vi "termo_main__.vi"() -> ()   [LabVIEW 2015]
doc: "Термометрия"
uses:
  <vilib>/NI/Modbus Library/API/Master/Modbus Master.lvclass
  Load and Save Controls_LV2009.llb/RWC_Actions.ctl
  <vilib>/Utility/error.llb/DialogType.ctl
  <vilib>/express/express arith-compare/Formula/XNode/ExpressFormulaBlockNode.xnode
panel:
  in  "счетчик":u16
  out "Связь с блоком":bool
  in  "Tab Control":enum32{"ИЗМЕРЕНИЯ", "НАСТРОЙКИ"}(tab)
  in  "3_ch_visible":bool=TRUE
  out "R2":dbl format="%.2f"
  out "R1":dbl format="%.2f"
  in  "2_ch_visible":bool=TRUE
  in  "1_ch_visible":bool=TRUE
  out "К 2":dbl format="%.2f"
  out "К 1":dbl format="%.2f"
  out "К 3":dbl format="%.2f"
  out "R3":dbl format="%.2f"
  in  "Т min":dbl=4.0 min=-10.0 max=350.0 step=0.1
  in  "Т max":dbl=350.0 min=2.0 max=500.0 step=0.1
  in  "Autoscale":bool=TRUE
  out "сек.":string="0"
  out "часы":string="0"
  in  "Добавить время":dbl(ring)=300.0 items=["10 сек."=10.0, "1 мин."=60.0, "5 мин."=300.0, "20 мин."=1200.0]
  out "мин.":string="1"
  in  "xScale +":bool
  in  "xScale -":bool
  in  "Сохранение в файл":bool
  in  "Buf_size":u16=10 min=1 max=128
  in  "SPS":T1(ring)=enum."5 SPS"
  in  "Пароль":string
  in  "настр. коэфф.":bool caption="Disconn"
  in  "Коэ 2":T2 caption="К 2" {"R0" format="%#_16g"; "k7" format="%#_16g"; "k6" format="%#_16g"; "k5" format="%#_16g"; "k4" format="%#_16g"; "k3" format="%#_16g"; "k2" format="%#_16g"; "k1" format="%#_16g"}
  in  "stop":bool
  in  "Коэ 1":T2 caption="К 1" {"R0" format="%#_16g"; "k7" format="%#_16g"; "k6" format="%#_16g"; "k5" format="%#_16g"; "k4" format="%#_16g"; "k3" format="%#_16g"; "k2" format="%#_16g"; "k1" format="%#_16g"}
  in  "GraphLookB":bool
  in  "IP":string
  in  "Порт":u16
  in  "Коэ 3":T2 caption="К 3" {"R0" format="%#_16g"; "k7" format="%#_16g"; "k6" format="%#_16g"; "k5" format="%#_16g"; "k4" format="%#_16g"; "k3" format="%#_16g"; "k2" format="%#_16g"; "k1" format="%#_16g"}
  out "Path":string
  in  "интервал сохр.":u16=10 min=1 max=3600 step=1
  out "Сутки":string
  in  "Запись в файл":bool
  out "File header exist?":bool caption="Disconn"
  in  "ADC_dyn_range":T3(ring)=enum."± 0.625 В"
  out "refnum out":refnum<file>
  out "Graphs T":dynamicdata(graph) caption="ТЕМПЕРАТУРА, К"
  out "Связь":refnum<class "Modbus Master.lvclass">
  in  "Buf_size":u8=1 min=1 max=128
  in  "SPS":T1(ring)
  out "Расположение файла":path
  # "Т [K]"
  # "R [Ом]"
  # ":"
  # ":"
  # "Шкала Т"
  # "id 100"
  # "Скорость измерений"
  # "Размер буфера усредн."
  # "SPS = Samples Per Second"
  # "сек."
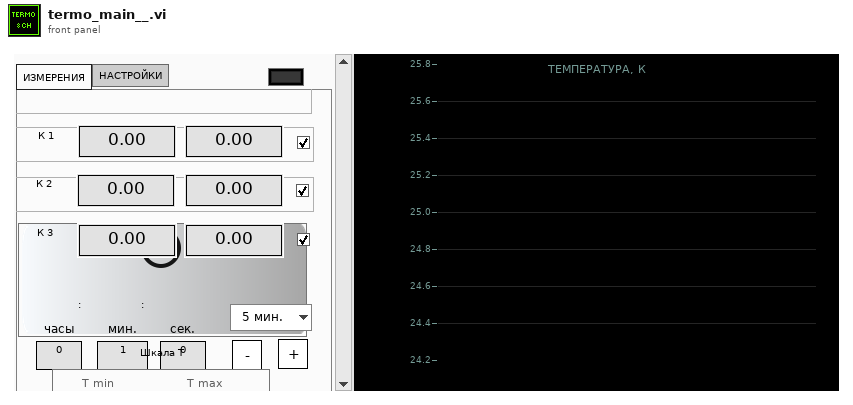
[diagram p1: front panel]
types:
  T1 = enum16{"2,5 SPS", "5 SPS", "10 SPS", "25 SPS", "50 SPS", "100 SPS", "500 SPS", "1 kSPS"}
  T2 = cluster{"k1":ext, "k2":ext, "k3":ext, "k4":ext, "k5":ext, "k6":ext, "k7":ext, "R0":ext}
  T3 = enum16{"± 5 В", "± 2.5 В", "± 1.25 В", "± 0.625 В", "± 312.5 мВ", "± 156.25 мВ", "± 78.125 мВ"}
  T4 = typedef "DialogType.ctl" = u16
  T5 = typedef "RWC_Actions.ctl" = enum16{"Read", "Write", "Read and Create"}
  T6 = enum8{"Enabled", "Disabled", "Disabled and Grayed Out"}
  T7 = typedef "LVDateTimeRec.ctl" = cluster{"fractional second":dbl, "second":i32, "minute":i32, "hour":i32, "day of month":i32, "month":i32, "year":i32, "day of week":i32, "day of year":i32, "DST":i32}
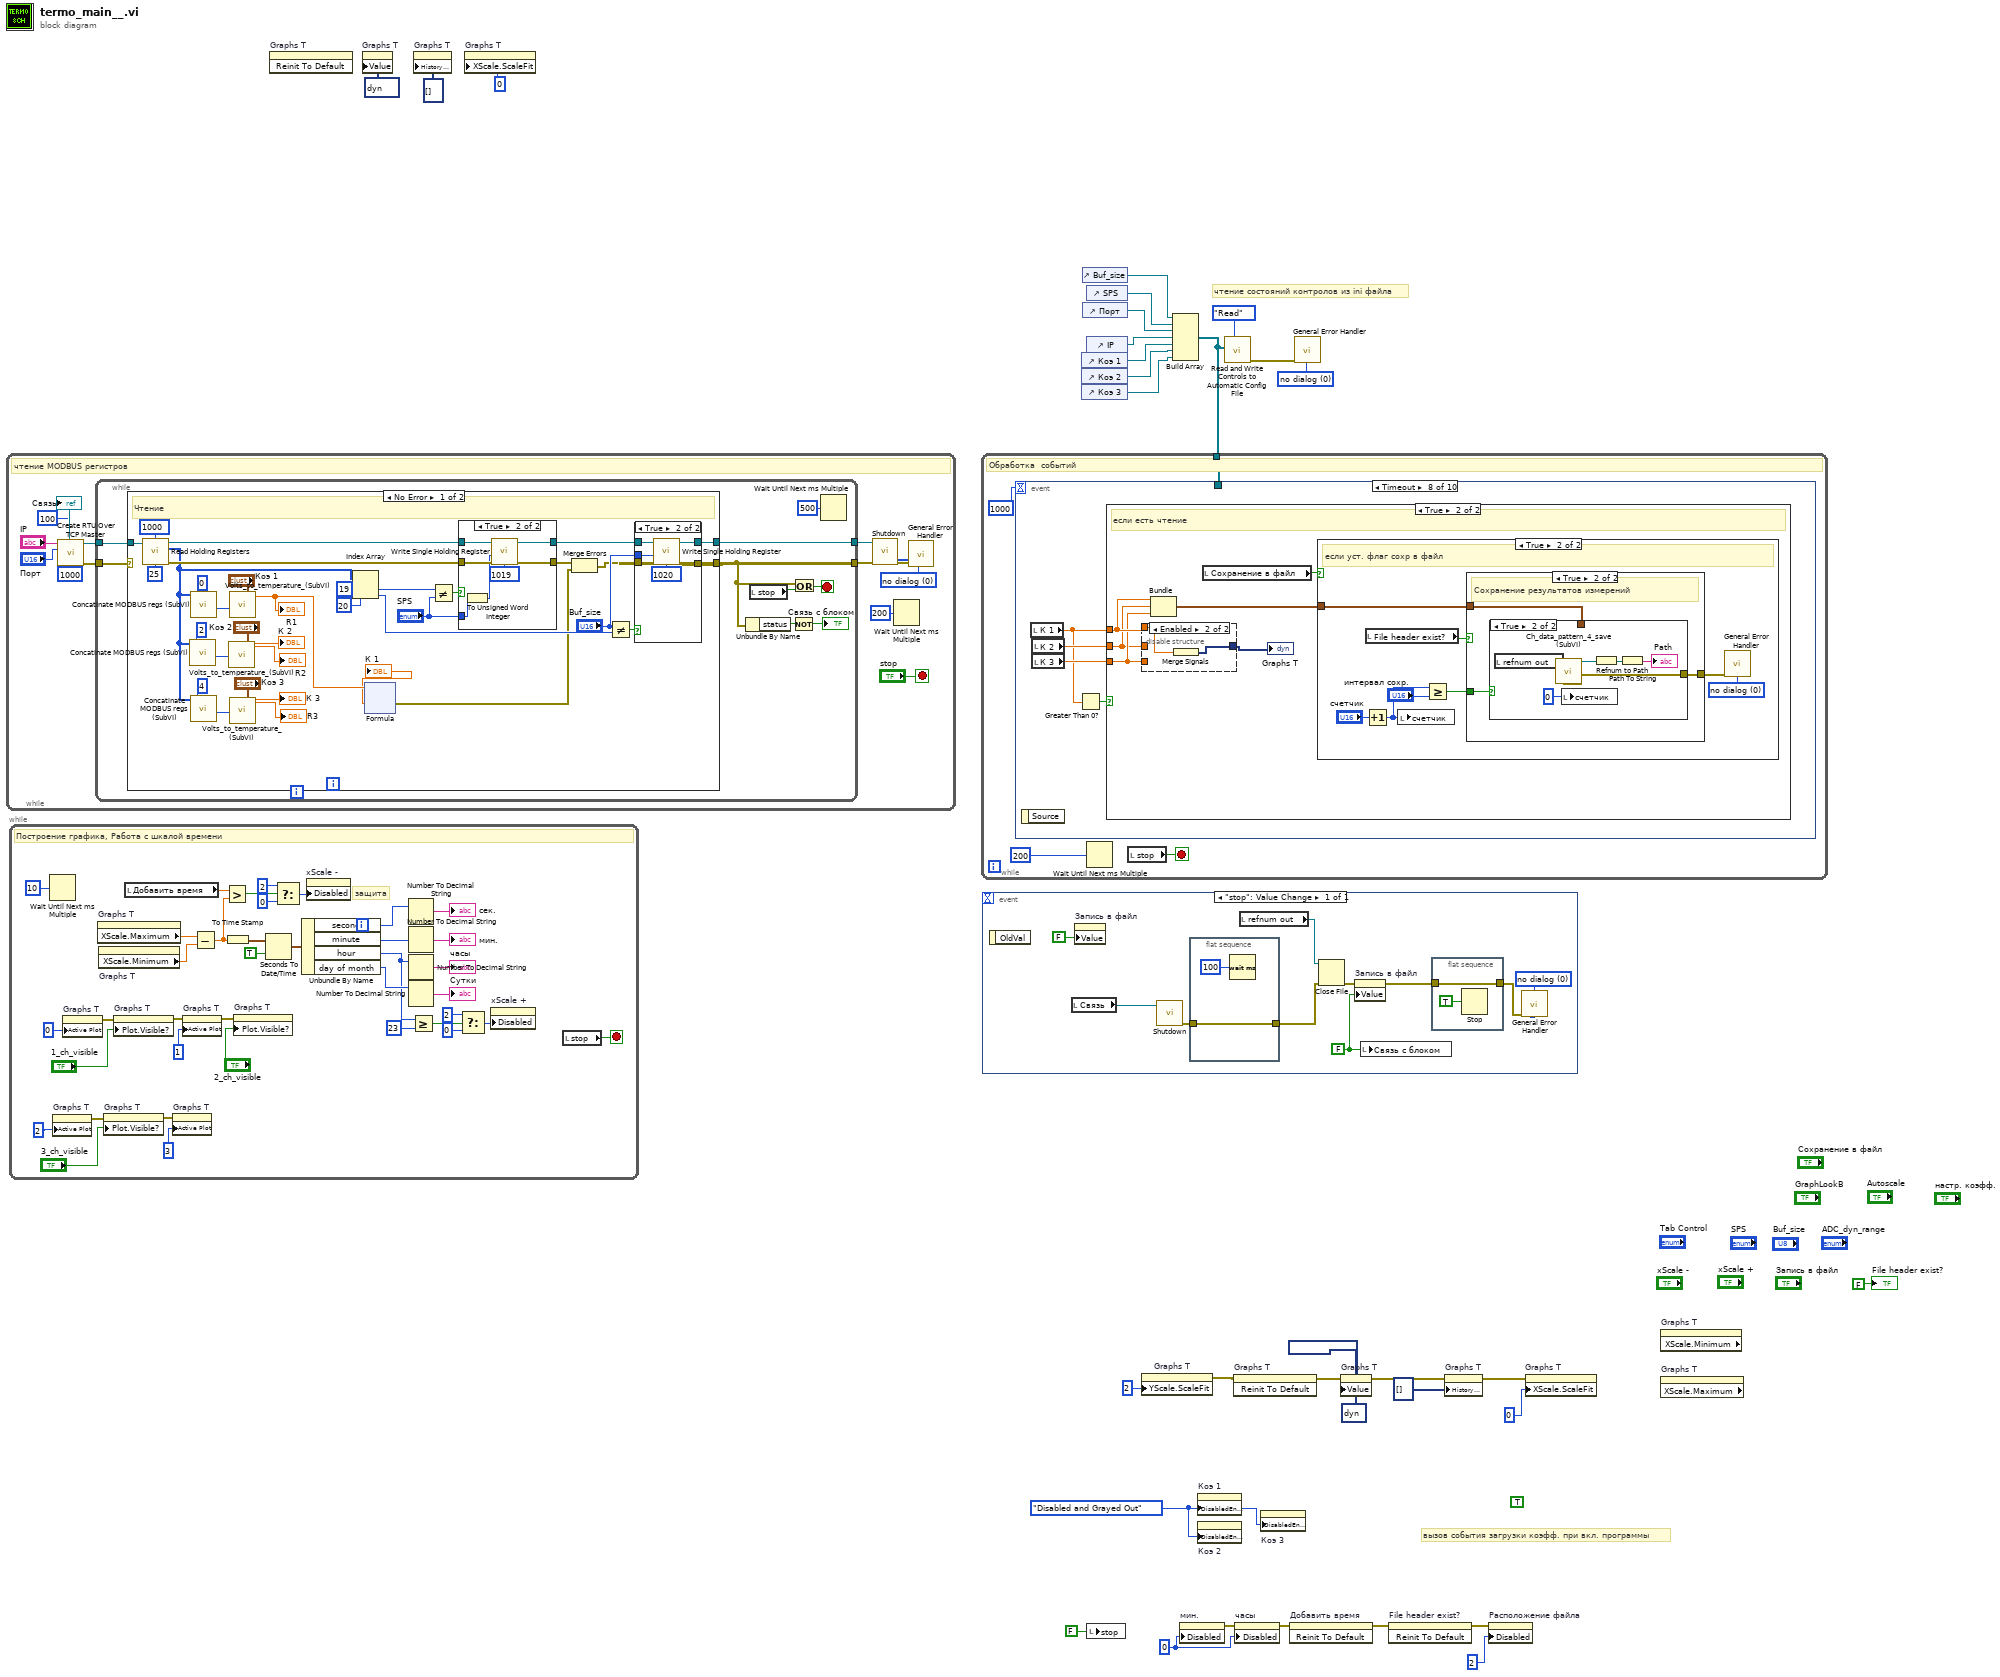
[diagram p0: block diagram]
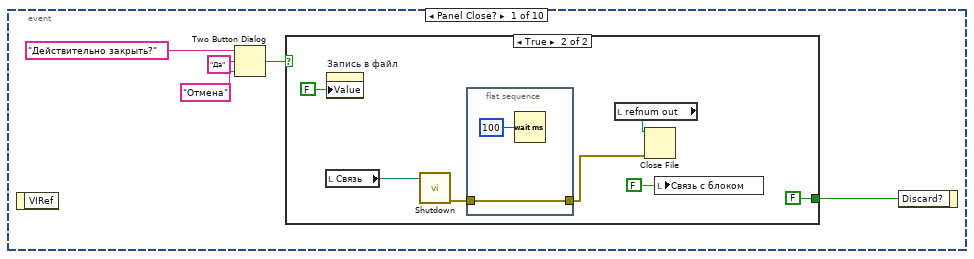
[diagram p2: hidden frame]
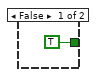
[diagram p3: hidden frame]
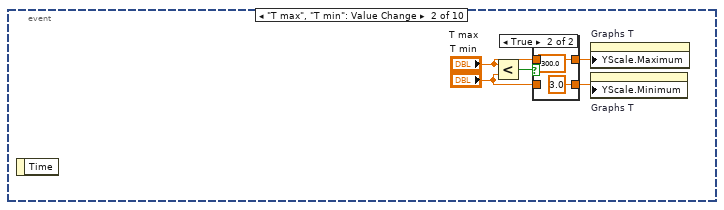
[diagram p4: hidden frame]
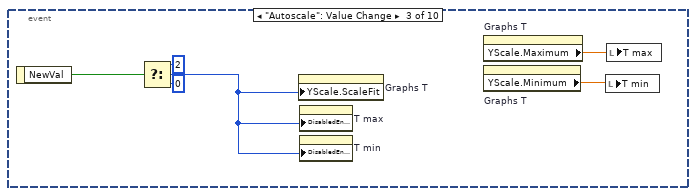
[diagram p6: hidden frame]
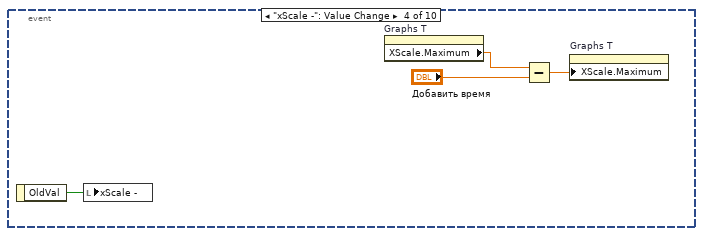
[diagram p7: hidden frame]
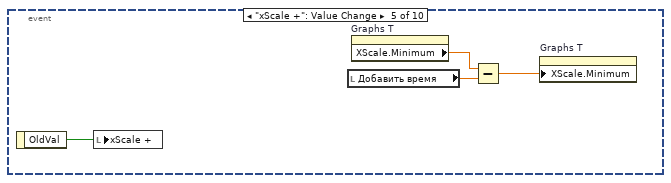
[diagram p8: hidden frame]
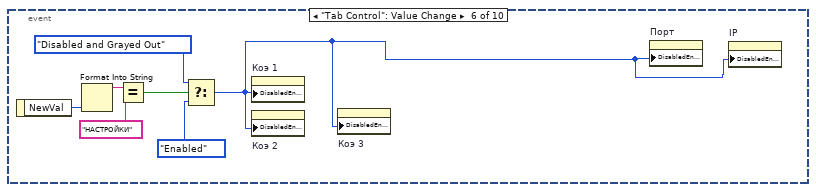
[diagram p9: hidden frame]
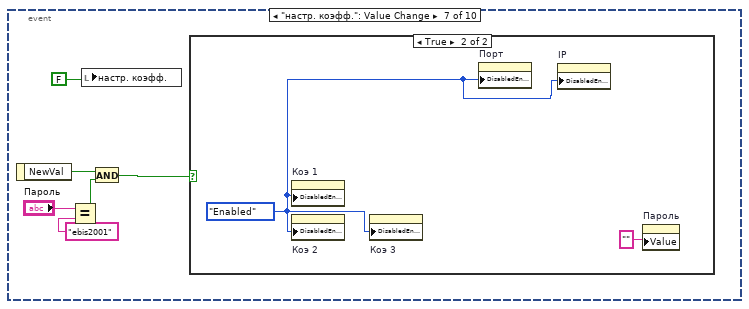
[diagram p10: hidden frame]
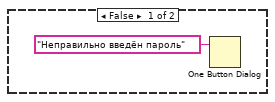
[diagram p11: hidden frame]
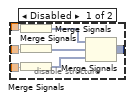
[diagram p13: hidden frame]
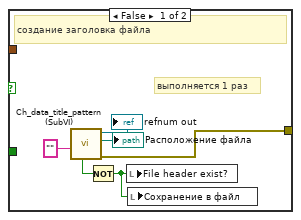
[diagram p15: hidden frame]
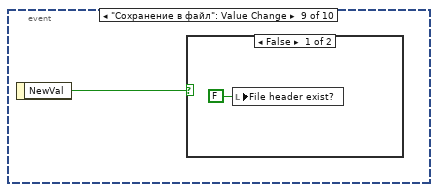
[diagram p17: hidden frame]
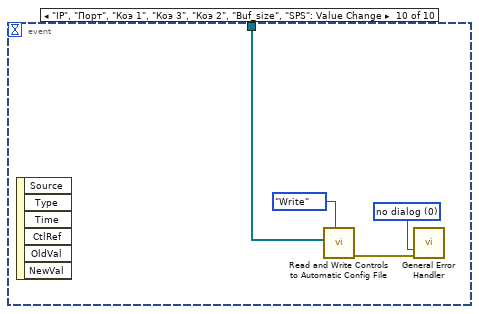
[diagram p19: hidden frame]
diagram:
  w12 = T4 0 items=["no dialog", "OK message", "continue or stop message", "OK message + warnings", "continue/stop + warnings"] ("type of dialog (OK msg:1)")
  (unwired) TRUE ("Value (Signaling)")
  w15 = T6."Disabled and Grayed Out" ("Disabled")
  w30 = u8 0 ("Disabled")
  # "чтение состояний контролов из ini файла"
  # "вызов события загрузки коэфф. при вкл. программы"
  n1 = while {
    stop <- "stop" stop-if-true
    w33 = T4 0 items=["no dialog", "OK message", "continue or stop message", "OK message + warnings", "continue/stop + warnings"] ("type of dialog (OK msg:1)")
    # "чтение MODBUS регистров"
    n2 = call "Create RTU Over TCP Master.vi"("unit ID"=u8 100, "connect timeout ms"=1000, "port (502)"="Порт", "address"="IP") -> ("error out"=w37:errorcluster, "TCP master instance"=w38:refnum<class "Modbus Master.lvclass">)  [unwired: 6 in]
    "Связь" <- w38
    n3 = while {
      tunnel: w38 -> [w52]
      tunnel: w37 -> [w51]
      tunnel: [w45] -> w36
      tunnel: [w50] -> w35
      stop <- w48 stop-if-true
      n4 = case shown="No Error" w51 {
        selector: w51 -> [_ w117]
        tunnel: w52 -> [w85 w118]
        tunnel: [w69 w117] -> w45
        tunnel: [w70 w118] -> w50
        frame No Error {
          # "Чтение"
          n5 = call-dynamic "Read Holding Registers.vi"("number of inputs"=u16 25, "starting address"=u16 1000, "Modbus master in"=w85) -> ("error out"=w67:errorcluster, "register values"=w66:u16[], "Modbus master out"=w68:refnum<class "Modbus Master.lvclass">)  [unwired: 6 in]
          n6 = call "Concatinate MODBUS regs (SubVI).vi"("LSB reg num"=u16 2, "registers array in"=w66) -> ("register data"=w80:i32)  [unwired: 8 in, 1 out]
          n7 = call "Concatinate MODBUS regs (SubVI).vi"("LSB reg num"=u16 0, "registers array in"=w66) -> ("register data"=w82:i32)  [unwired: 8 in, 1 out]
          n8 = call "Concatinate MODBUS regs (SubVI).vi"("LSB reg num"=u16 4, "registers array in"=w66) -> ("register data"=w73:i32)  [unwired: 8 in, 1 out]
          n9 = call "Volts_to_temperature_(SubVI).vi"("Resistance"=w80, "koeff. cluster"="Коэ 2") -> ("T solvation"=→"К 2":dbl, "meas_voltage"=→"R2":dbl)  [unwired: 21 in, 3 out]
          n10 = call "Volts_to_temperature_(SubVI).vi"("Resistance"=w82, "koeff. cluster"="Коэ 1") -> ("meas_voltage"=w57:dbl)  [unwired: 21 in, 4 out]
          "R1" <- w57
          n11 = call "Volts_to_temperature_(SubVI).vi"("Resistance"=w73, "koeff. cluster"="Коэ 3") -> ("T solvation"=→"К 3":dbl, "meas_voltage"=→"R3":dbl)  [unwired: 21 in, 3 out]
          n12 = Index Array(array=w66, index #1=19 ("index"), index #2=20 ("index")) -> (element #1=w65:u16, element #2=w59:u16)
          n13 = xnode "Formula"("R"=w57) -> ("Result"=→"К 1":ext, "error out"=w53:errorcluster)  [unwired: 2 in]
          n14 = Not Equal?(x=w65, y="SPS") -> (x != y?=w64:bool)
          n15 = case shown="True" w64 {
            tunnel: w68 -> [w107 w114]
            tunnel: w67 -> [w106 w113]
            tunnel: [w107 w111] -> w71
            tunnel: [w106 w110] -> w55
            tunnel: "SPS" -> [_ w109]
            frame False {
            }
            frame True {
              n16 = To Unsigned Word Integer(number=w109) -> (unsigned 16bit integer=w108:u16)
              n17 = call-dynamic "Write Single Holding Register.vi"("error in"=w113, "register to write"=w108, "address"=u16 1019 ("starting address"), "Modbus master in"=w114) -> ("error out"=w110:errorcluster, "Modbus master out"=w111:refnum<class "Modbus Master.lvclass">)  [unwired: 6 in]
            }
          }
          n18 = Merge Errors(w55, w53) -> (w54:errorcluster)
          n19 = Not Equal?(x="Buf_size", y=w59) -> (x != y?=w60:bool)
          n20 = case shown="True" w60 {
            tunnel: w71 -> [w99 w105]
            tunnel: w54 -> [w98 w104]
            tunnel: [w99 w102] -> w70
            tunnel: [w98 w101] -> w69
            tunnel: "Buf_size" -> [_ w100]
            frame False {
            }
            frame True {
              n21 = call-dynamic "Write Single Holding Register.vi"("error in"=w104, "register to write"=w100, "address"=u16 1020 ("starting address"), "Modbus master in"=w105) -> ("error out"=w101:errorcluster, "Modbus master out"=w102:refnum<class "Modbus Master.lvclass">)  [unwired: 6 in]
            }
          }
        }
        frame Error {
          w115 = -1.0 ("R1")
          w116 = -1.0 ("R1")
          n22 = local write "R1"(w115) -> ()
          n23 = local write "R2"(w115) -> ()
          n24 = local write "R3"(w115) -> ()
          n25 = local write "К 1"(w116) -> ()
          n26 = local write "К 3"(w116) -> ()
          n27 = local write "К 2"(w116) -> ()
        }
      }
      n28 = Unbundle By Name(w45) -> ("status"=w47:bool)
      n29 = local read "stop"() -> (w49:bool)
      n30 = Not(x=w47) -> (.not. x?=→"Связь с блоком":bool)
      n31 = Or(x=w45, y=w49) -> (x .or. y?=w48:bool)
      n32 = Wait Until Next ms Multiple(millisecond multiple=u32 500) -> ()  [unwired: 1 out]
    }
    n33 = call-dynamic "Shutdown.vi"("error in"=w36, "Modbus master in"=w35) -> ("error out"=w34:errorcluster)  [unwired: 9 in]
    n34 = Wait Until Next ms Multiple(millisecond multiple=u32 200) -> ()  [unwired: 1 out]
    n35 = call <vilib>:"General Error Handler.vi"("type of dialog (OK msg:1)"=w33, "error in (no error)"=w34) -> ()  [unwired: 1 in, 13 out]
  }
  n36 = while {
    stop <- w156 stop-if-true
    # "защита"
    # "Построение графика, Работа с шкалой времени"
    n37 = Wait Until Next ms Multiple(millisecond multiple=u32 10) -> ()  [unwired: 1 out]
    n38 = property on="Graphs T" class="WFChart (strict)"("Active Plot"=u32 2) -> (error out=w123:errorcluster)  [unwired: 2 in, 1 out]
    n39 = property on="Graphs T" class="WFChart (strict)"("Active Plot"=u32 0) -> (error out=w124:errorcluster)  [unwired: 2 in, 1 out]
    n40 = property on="Graphs T" class="WFChart (strict)"() -> ("XScale.Maximum"=w132:dbl)  [unwired: 2 in, 2 out]
    n41 = property on="Graphs T" class="WFChart (strict)"() -> ("XScale.Minimum"=w131:dbl)  [unwired: 2 in, 2 out]
    n42 = property on="Graphs T" class="WFChart (strict)"(error in=w123, "Plot.Visible?"="3_ch_visible") -> (error out=w119:errorcluster)  [unwired: 1 in, 1 out]
    n43 = property on="Graphs T" class="WFChart (strict)"(error in=w124, "Plot.Visible?"="1_ch_visible") -> (error out=w129:errorcluster)  [unwired: 1 in, 1 out]
    n44 = local read "Добавить время"() -> (w155:dbl)
    n45 = property on="Graphs T" class="WFChart (strict)"(error in=w119, "Active Plot"=u32 3) -> ()  [unwired: 1 in, 2 out]
    n46 = property on="Graphs T" class="WFChart (strict)"(error in=w129, "Active Plot"=u32 1) -> (error out=w127:errorcluster)  [unwired: 1 in, 1 out]
    n47 = Subtract(x=w132, y=w131) -> (x-y=w145:dbl)
    n48 = Greater?(x=w155, y=w145) -> (0:w138:bool)
    n49 = To Time Stamp(1:w145) -> (0:w153:timestamp)
    n50 = property on="Graphs T" class="WFChart (strict)"(error in=w127, "Plot.Visible?"="2_ch_visible") -> ()  [unwired: 1 in, 2 out]
    n51 = Seconds To Date/Time(time stamp (now)=w153, to UTC (F)=TRUE) -> (date time rec=w152:T7)
    n52 = Select(t=u8 2 ("Disabled"), s=w138, f=u8 0 ("Disabled")) -> (s? t:f=w141:u8)
    n53 = Unbundle By Name(w152) -> ("second"=w151:i32, "minute"=w150:i32, "hour"=w143:i32, "day of month"=w149:i32)
    n54 = property on="xScale -" class="Bool (strict)"("Disabled"=w141) -> ()  [unwired: 2 in, 2 out]
    n55 = Number To Decimal String(number=w151) -> (decimal integer string=→"сек.":string)  [unwired: 1 out]
    n56 = Number To Decimal String(number=w150) -> (decimal integer string=→"мин.":string)  [unwired: 1 out]
    n57 = Number To Decimal String(number=w143) -> (decimal integer string=→"часы":string)  [unwired: 1 out]
    n58 = Number To Decimal String(number=w149) -> (decimal integer string=→"Сутки":string)  [unwired: 1 out]
    n59 = Greater Or Equal?(x=w143, y=23) -> (x >= y?=w134:bool)
    n60 = Select(t=u8 2 ("Disabled"), s=w134, f=u8 0 ("Disabled")) -> (s? t:f=w137:u8)
    n61 = property on="xScale +" class="Bool (strict)"("Disabled"=w137) -> ()  [unwired: 2 in, 2 out]
    n62 = local read "stop"() -> (w156:bool)
  }
  n63 = invoke on="Graphs T" class="WFChart (strict)" method="Reinit To Default"() -> ()  [unwired: 3 in, 3 out]
  n64 = property on="Graphs T" class="WFChart (strict)"("Value"=dynamicdata [{"t0"=timestamp(3465273261.7246556 s since 1904-01-01), "dt"=1.0, "Y"=[0.1931097262457384]}, {"t0"=timestamp(3465273261.7246556 s since 1904-01-01), "dt"=1.0, "Y"=[0.3594116459482981]}, {"t0"=timestamp(3465273261.7246556 s since 1904-01-01), "dt"=1.0, "Y"=[0.8898205452798131]}, {"t0"=timestamp(3465273261.7246556 s since 1904-01-01), "dt"=1.0, "Y"=[0.747699236883661]}] ("Graphs")) -> ()  [unwired: 2 in, 2 out]
  n65 = property on="Graphs T" class="WFChart (strict)"("History Data"=dynamicdata[] []) -> ()  [unwired: 2 in, 2 out]
  n66 = property on="Graphs T" class="WFChart (strict)"("XScale.ScaleFit"=u8 0 ("Y Scale.Scale Fit")) -> ()  [unwired: 2 in, 2 out]
  n67 = event shown="[0] \"stop\": Value Change" {
    selector: _ -> [_]
    dyn-events: _ -> [_]
    timeout: _ -> [_]
    event "stop": Value Change {
      w160 = T4 0 items=["no dialog", "OK message", "continue or stop message", "OK message + warnings", "continue/stop + warnings"] ("type of dialog (OK msg:1)")
      w157 = FALSE ("Запись в файл")
      n68 = event-data() -> ()  [unwired: 1 in, 1 out]
      n69 = local read "Связь"() -> (w162:refnum<class "Modbus Master.lvclass">)
      n70 = property on="Запись в файл" class="Bool (strict)"("Value"=FALSE ("Запись в файл")) -> ()  [unwired: 2 in, 2 out]
      n71 = call-dynamic "Shutdown.vi"("Modbus master in"=w162) -> ("error out"=w161:errorcluster)  [unwired: 10 in]
      n72 = flat-sequence {
        tunnel: w161 -> [w169]
        tunnel: [w169] -> w158
        frame #0 {
          n73 = Wait (ms)(milliseconds to wait=u32 100) -> ()  [unwired: 1 out]
        }
      }
      n74 = local read "refnum out"() -> (w165:refnum<file>)
      n75 = Close File(refnum=w165, error in=w158) -> (error out=w164:errorcluster)  [unwired: 1 out]
      n76 = property on="Запись в файл" class="Bool (strict)"(error in=w164, "Value"=w157) -> (error out=w163:errorcluster)  [unwired: 1 in, 1 out]
      n77 = local write "Связь с блоком"(w157) -> ()
      n78 = flat-sequence {
        tunnel: w163 -> [w168]
        tunnel: [w168] -> w159
        frame #0 {
          n79 = Stop(stop? (T)=TRUE) -> ()
        }
      }
      n80 = call <vilib>:"General Error Handler.vi"("error in (no error)"=w159, "[exception action] (none:0)"=w160) -> ()  [unwired: 2 in, 12 out]
    }
  }
  n81 = control-ref of="Коэ 1"() -> (w6:refnum<vi>)
  n82 = control-ref of="Коэ 2"() -> (w5:refnum<vi>)
  n83 = control-ref of="Коэ 3"() -> (w4:refnum<vi>)
  n84 = control-ref of="Buf_size"() -> (w8:refnum<vi>)
  n85 = control-ref of="Порт"() -> (w11:refnum<vi>)
  n86 = control-ref of="SPS"() -> (w9:refnum<vi>)
  n87 = control-ref of="IP"() -> (w7:refnum<vi>)
  n88 = local write "stop"(FALSE ("Boolean")) -> ()
  n89 = property on="Graphs T" class="WFChart (strict)"("YScale.ScaleFit"=u8 2 ("Y Scale.Scale Fit")) -> (error out=w23:errorcluster)  [unwired: 2 in, 1 out]
  n90 = Build Array(w8, w9, w11, w7, w6, w5, w4) -> (w10:refnum<vi>[])
  n91 = while {
    tunnel: w10 -> [w171]
    stop <- w173 stop-if-true
    # "Обработка  событий"
    n92 = event shown="[7] Timeout" {
      selector: _ -> [_ _ _ _ _ _ _ _ _ _]
      dyn-events: _ -> [_ _ _ _ _ _ _ _ _ _]
      timeout: 1000 -> [_ _ _ _ _ _ _ _ _ _]
      tunnel: w171 -> [_ _ _ _ _ _ _ _ _ w272]
      event Panel Close? {
        n93 = event-data() -> ()  [unwired: 2 out]
        n94 = Two Button Dialog(message="Действительно закрыть?", 1:"Отмена" ("T button name (\"OK\")"), 2:"Да" ("T button name (\"OK\")")) -> (T button?=w179:bool)
        n95 = case shown="True" w179 {
          tunnel: [TRUE ("Discard?") FALSE ("Discard?")] -> w175
          frame False {
          }
          frame True {
            n96 = local read "Связь"() -> (w184:refnum<class "Modbus Master.lvclass">)
            n97 = property on="Запись в файл" class="Bool (strict)"("Value"=FALSE ("Запись в файл")) -> ()  [unwired: 2 in, 2 out]
            n98 = call-dynamic "Shutdown.vi"("Modbus master in"=w184) -> ("error out"=w183:errorcluster)  [unwired: 10 in]
            n99 = flat-sequence {
              tunnel: w183 -> [w188]
              tunnel: [w188] -> w182
              frame #0 {
                n100 = Wait (ms)(milliseconds to wait=u32 100) -> ()  [unwired: 1 out]
              }
            }
            n101 = local read "refnum out"() -> (w186:refnum<file>)
            n102 = Close File(refnum=w186, error in=w182) -> ()  [unwired: 2 out]
            n103 = local write "Связь с блоком"(FALSE ("Связь с блоком 4")) -> ()
          }
        }
        n104 = event-data("Discard?"=w175) -> ()  [unwired: 1 in, 1 out]
      }
      event "Т max", "Т min": Value Change {
        n105 = event-data() -> ()  [unwired: 2 out]
        n106 = Less?(x="Т max", y="Т min") -> (x < y?=w194:bool)
        n107 = case shown="True" w194 {
          tunnel: [w195 300.0 ("x+1")] -> w192
          tunnel: [w196 3.0 ("x+1")] -> w193
          tunnel: "Т max" -> [w195 _]
          tunnel: "Т min" -> [w196 _]
          frame False {
          }
          frame True {
          }
        }
        n108 = property on="Graphs T" class="WFChart (strict)"("YScale.Maximum"=w192) -> ()  [unwired: 2 in, 2 out]
        n109 = property on="Graphs T" class="WFChart (strict)"("YScale.Minimum"=w193) -> ()  [unwired: 2 in, 2 out]
      }
      event "Autoscale": Value Change {
        n110 = event-data() -> ("NewVal"=w199:bool)  [unwired: 1 out]
        n111 = Select(t=u8 2 ("Y Scale.Scale Fit"), s=w199, f=u8 0 ("Y Scale.Scale Fit")) -> (s? t:f=w202:u8)
        n112 = property on="Graphs T" class="WFChart (strict)"("YScale.ScaleFit"=w202) -> ()  [unwired: 2 in, 2 out]
        n113 = property on="Т max" class="DigNum (strict)"("DisabledEnum"=w202) -> ()  [unwired: 2 in, 2 out]
        n114 = property on="Т min" class="DigNum (strict)"("DisabledEnum"=w202) -> ()  [unwired: 2 in, 2 out]
        n115 = property on="Graphs T" class="WFChart (strict)"() -> ("YScale.Maximum"=w204:dbl)  [unwired: 2 in, 2 out]
        n116 = property on="Graphs T" class="WFChart (strict)"() -> ("YScale.Minimum"=w203:dbl)  [unwired: 2 in, 2 out]
        n117 = local write "Т min"(w203) -> ()
        n118 = local write "Т max"(w204) -> ()
      }
      event "xScale -": Value Change {
        n119 = event-data() -> ("OldVal"=w208:bool)  [unwired: 1 out]
        n120 = local write "xScale -"(w208) -> ()
        n121 = property on="Graphs T" class="WFChart (strict)"() -> ("XScale.Maximum"=w206:dbl)  [unwired: 2 in, 2 out]
        n122 = Subtract(x=w206, y="Добавить время") -> (x-y=w205:dbl)
        n123 = property on="Graphs T" class="WFChart (strict)"("XScale.Maximum"=w205) -> ()  [unwired: 2 in, 2 out]
      }
      event "xScale +": Value Change {
        n124 = event-data() -> ("OldVal"=w212:bool)  [unwired: 1 out]
        n125 = local write "xScale +"(w212) -> ()
        n126 = local read "Добавить время"() -> (w211:dbl)
        n127 = property on="Graphs T" class="WFChart (strict)"() -> ("XScale.Minimum"=w210:dbl)  [unwired: 2 in, 2 out]
        n128 = Subtract(x=w210, y=w211) -> (x-y=w209:dbl)
        n129 = property on="Graphs T" class="WFChart (strict)"("XScale.Minimum"=w209) -> ()  [unwired: 2 in, 2 out]
      }
      event "Tab Control": Value Change {
        n130 = event-data() -> ("NewVal"=w219:enum32{"ИЗМЕРЕНИЯ", "НАСТРОЙКИ"})  [unwired: 1 out]
        n131 = Format Into String(w219) -> (resulting string=w218:string)  [unwired: 3 in, 1 out]
        n132 = Equal?(x=w218, y="НАСТРОЙКИ") -> (x = y?=w216:bool)
        n133 = Select(t=T6."Disabled and Grayed Out" ("Disabled"), s=w216, f=T6."Enabled" ("Disabled")) -> (s? t:f=w213:T6)
        n134 = property on="Коэ 1" class="Clust (strict)"("DisabledEnum"=w213) -> ()  [unwired: 2 in, 2 out]
        n135 = property on="Коэ 2" class="Clust (strict)"("DisabledEnum"=w213) -> ()  [unwired: 2 in, 2 out]
        n136 = property on="Коэ 3" class="Clust (strict)"("DisabledEnum"=w213) -> ()  [unwired: 2 in, 2 out]
        n137 = property on="Порт" class="DigNum (strict)"("DisabledEnum"=w213) -> ()  [unwired: 2 in, 2 out]
        n138 = property on="IP" class="Str"("DisabledEnum"=w213) -> ()  [unwired: 2 in, 2 out]
      }
      event "настр. коэфф.": Value Change {
        n139 = event-data() -> ("NewVal"=w225:bool)  [unwired: 1 out]
        n140 = Equal?(x="Пароль", y="ebis2001") -> (x = y?=w222:bool)
        n141 = local write "настр. коэфф."(FALSE ("насстр. коэфф.")) -> ()
        n142 = And(x=w225, y=w222) -> (x .and. y?=w221:bool)
        n143 = case shown="True" w221 {
          frame False {
            n144 = One Button Dialog(message="Неправильно введён пароль") -> ()  [unwired: 1 in, 1 out]
          }
          frame True {
            w227 = T6."Enabled" ("Disabled")
            n145 = property on="Коэ 1" class="Clust (strict)"("DisabledEnum"=w227) -> ()  [unwired: 2 in, 2 out]
            n146 = property on="Коэ 2" class="Clust (strict)"("DisabledEnum"=w227) -> ()  [unwired: 2 in, 2 out]
            n147 = property on="Коэ 3" class="Clust (strict)"("DisabledEnum"=w227) -> ()  [unwired: 2 in, 2 out]
            n148 = property on="Порт" class="DigNum (strict)"("DisabledEnum"=w227) -> ()  [unwired: 2 in, 2 out]
            n149 = property on="IP" class="Str"("DisabledEnum"=w227) -> ()  [unwired: 2 in, 2 out]
            n150 = property on="Пароль" class="Str"("Value"="" ("Пароль")) -> ()  [unwired: 2 in, 2 out]
          }
        }
      }
      event Timeout {
        n151 = event-data() -> ()  [unwired: 2 out]
        n152 = local read "К 1"() -> (w229:dbl)
        n153 = local read "К 2"() -> (w232:dbl)
        n154 = local read "К 3"() -> (w230:dbl)
        n155 = Greater Than 0?(x=w229) -> (x > 0?=w231:bool)
        n156 = case shown="True" w231 {
          tunnel: w229 -> [_ w237]
          tunnel: w230 -> [_ w236]
          tunnel: w232 -> [_ w234]
          frame False {
          }
          frame True {
            # "если есть чтение"
            n157 = disable-structure shown="Enabled" {
              disable-tunnel: [w242 w246] -> w238
              disable-tunnel: w237 -> [w241 w247]
              disable-tunnel: w236 -> [w240 _]
              disable-tunnel: w234 -> [w239 _]
              frame Disabled {
                n158 = Merge Signals(w241) -> (w245:dynamicdata)
                n159 = Merge Signals(w239) -> (w244:dynamicdata)
                n160 = Merge Signals(w240) -> (w243:dynamicdata)
                n161 = Merge Signals(w245, w244, w243) -> (w242:dynamicdata)
              }
              frame Enabled {
                n162 = Merge Signals(w247) -> (w246:dynamicdata)
              }
            }
            "Graphs T" <- w238
            n163 = Bundle("К 1"=w237, "К 2"=w234, "К 3"=w236) -> (w235:cluster{"К 1":dbl, "К 2":dbl, "К 3":dbl})  [unwired: 1 in]
            n164 = local read "Сохранение в файл"() -> (w233:bool)
            n165 = case shown="True" w233 {
              tunnel: w235 -> [_ w255]
              frame False {
              }
              frame True {
                w254 = T4 0 items=["no dialog", "OK message", "continue or stop message", "OK message + warnings", "continue/stop + warnings"] ("type of dialog (OK msg:1)")
                # "если уст. флаг сохр в файл"
                n166 = Increment(x="счетчик") -> (x+1=w251:u16)
                n167 = local read "File header exist?"() -> (w249:bool)
                n168 = local write "счетчик"(w251) -> ()
                n169 = Greater Or Equal?(x=w251, y="интервал сохр.") -> (x >= y?=w250:bool)
                n170 = case shown="True" w249 {
                  tunnel: w255 -> [_ w264]
                  tunnel: [w258 w263] -> w253
                  tunnel: w250 -> [_ w262]
                  frame False {
                    # "выполняется 1 раз"
                    # "создание заголовка файла"
                    n171 = call "Ch_data_title_pattern (SubVI).vi"("Единица измерений"="") -> ("error out"=w258:errorcluster, "Path"=→"Расположение файла":path, "Byte Stream File out"=→"refnum out":refnum<file>, "cancelled"=w257:bool)  [unwired: 7 in]
                    n172 = Not(x=w257) -> (.not. x?=w256:bool)
                    n173 = local write "File header exist?"(w256) -> ()
                    n174 = local write "Сохранение в файл"(w256) -> ()
                  }
                  frame True {
                    # "Сохранение результатов измерений"
                    n175 = case shown="True" w262 {
                      tunnel: w264 -> [_ _]
                      tunnel: [_ w265] -> w263
                      frame False {
                      }
                      frame True {
                        n176 = local read "refnum out"() -> (w269:refnum<file>)
                        n177 = call "Ch_data_pattern_4_save (SubVI).vi"() -> ("error out"=w265:errorcluster)  [unwired: 27 in]
                        n178 = local write "счетчик"(u8 0 ("счетчик")) -> ()
                        n179 = Refnum to Path(1:w269) -> (0:w268:path)
                        n180 = Path To String(path=w268) -> (string=→"Path":string)
                      }
                    }
                  }
                }
                n181 = call <vilib>:"General Error Handler.vi"("type of dialog (OK msg:1)"=w254, "error in (no error)"=w253) -> ()  [unwired: 1 in, 13 out]
              }
            }
          }
        }
      }
      event "Сохранение в файл": Value Change {
        n182 = event-data() -> ("NewVal"=w270:bool)  [unwired: 1 out]
        n183 = case shown="False" w270 {
          frame False {
            n184 = local write "File header exist?"(FALSE ("File header exist?")) -> ()
          }
          frame True {
          }
        }
      }
      event "IP", "Порт", "Коэ 1", "Коэ 3", "Коэ 2", "Buf_size", "SPS": Value Change {
        w275 = T4 0 items=["no dialog", "OK message", "continue or stop message", "OK message + warnings", "continue/stop + warnings"] ("type of dialog (OK msg:1)")
        n185 = event-data() -> ()  [unwired: 7 out]
        n186 = call "Read and Write Controls to Automatic Config File.vi"("Action"=RWC_Actions."Write", "Control References"=w272) -> ("error out"=w274:errorcluster)  [unwired: 9 in]
        n187 = call <vilib>:"General Error Handler.vi"("type of dialog (OK msg:1)"=w275, "error in (no error)"=w274) -> ()  [unwired: 1 in, 13 out]
      }
    }
    n188 = Wait Until Next ms Multiple(millisecond multiple=u32 200) -> ()  [unwired: 1 out]
    n189 = local read "stop"() -> (w173:bool)
  }
  n190 = property on="мин." class="Str"("Disabled"=w30) -> (error out=w29:errorcluster)  [unwired: 2 in, 1 out]
  n191 = property on="Коэ 1" class="Clust (strict)"("DisabledEnum"=w15) -> ()  [unwired: 2 in, 2 out]
  n192 = property on="Коэ 2" class="Clust (strict)"("DisabledEnum"=w15) -> ()  [unwired: 2 in, 2 out]
  n193 = call "Read and Write Controls to Automatic Config File.vi"("Action"=RWC_Actions."Read", "Control References"=w10) -> ("error out"=w13:errorcluster)  [unwired: 9 in]
  n194 = invoke on="Graphs T" class="WFChart (strict)" method="Reinit To Default"(error in=w23) -> (error out=w19:errorcluster)  [unwired: 2 in, 2 out]
  n195 = property on="часы" class="Str"(error in=w29, "Disabled"=w30) -> (error out=w28:errorcluster)  [unwired: 1 in, 1 out]
  n196 = property on="Коэ 3" class="Clust (strict)"("DisabledEnum"=w15) -> ()  [unwired: 2 in, 2 out]
  n197 = invoke on="Добавить время" class="Ring (strict)" method="Reinit To Default"(error in=w28) -> (error out=w26:errorcluster)  [unwired: 2 in, 2 out]
  n198 = call <vilib>:"General Error Handler.vi"("type of dialog (OK msg:1)"=w12, "error in (no error)"=w13) -> ()  [unwired: 1 in, 13 out]
  n199 = property on="Graphs T" class="WFChart (strict)"(error in=w19, "Value"=dynamicdata [{"t0"=timestamp(3465273261.7246556 s since 1904-01-01), "dt"=1.0, "Y"=[0.1931097262457384]}, {"t0"=timestamp(3465273261.7246556 s since 1904-01-01), "dt"=1.0, "Y"=[0.3594116459482981]}, {"t0"=timestamp(3465273261.7246556 s since 1904-01-01), "dt"=1.0, "Y"=[0.8898205452798131]}, {"t0"=timestamp(3465273261.7246556 s since 1904-01-01), "dt"=1.0, "Y"=[0.747699236883661]}] ("Graphs")) -> (error out=w20:errorcluster)  [unwired: 1 in, 1 out]
  n200 = invoke on="File header exist?" class="Bool (strict)" method="Reinit To Default"(error in=w26) -> (error out=w27:errorcluster)  [unwired: 2 in, 2 out]
  n201 = property on="Graphs T" class="WFChart (strict)"(error in=w20, "History Data"=dynamicdata[] []) -> (error out=w17:errorcluster)  [unwired: 1 in, 1 out]
  n202 = property on="Расположение файла" class="Path"(error in=w27, "Disabled"=u8 2) -> ()  [unwired: 1 in, 2 out]
  n203 = property on="Graphs T" class="WFChart (strict)"(error in=w17, "XScale.ScaleFit"=u8 0 ("Y Scale.Scale Fit")) -> ()  [unwired: 1 in, 2 out]
  n204 = property on="Graphs T" class="WFChart (strict)" props=["XScale", "Minimum"]() -> ()  [unwired: 2 in, 3 out]
  n205 = property on="Graphs T" class="WFChart (strict)" props=["XScale", "Maximum"]() -> ()  [unwired: 2 in, 3 out]
  "File header exist?" <- FALSE ("flag1")
